vi "set_positions.vi"(7 "PicoMotor (in)":refnum<class "PicoMotor.lvclass">, 8 "error IO":errorcluster, 10 "enables":bool[](array[boolean]), 11 "set positions":i32[](array[numeric])) -> (0 "error out":errorcluster, 3 "PicoMotor":refnum<class "PicoMotor.lvclass">)   [LabVIEW 2013, in "PicoMotor.lvclass"]
uses:
  PicoMotor.lvclass
  PicoMotor.lvclass/PicoMotor.ctl
  Globals.vi
panel:
  out "enableds":bool[](array[boolean])
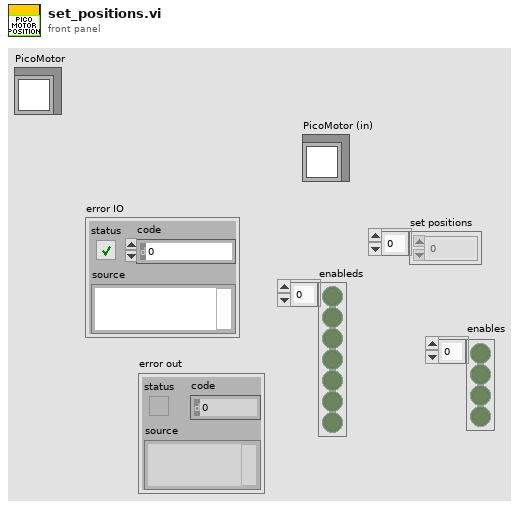
[diagram p1: front panel]
types:
  T1 = typedef "Experiment.lvclass/states.ctl" = enum16{"run", "pause", "shutdown gracefully", "halt immediately", "waiting for connection", "waiting for command"}
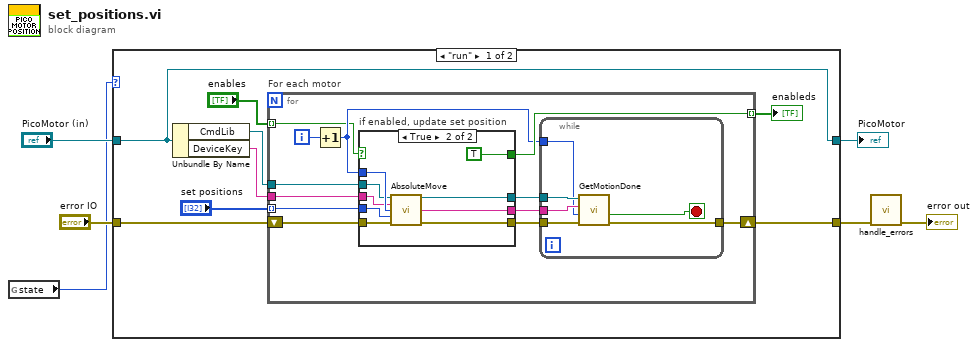
[diagram p0: block diagram]
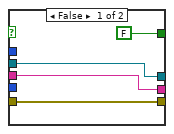
[diagram p2: hidden frame]
diagram:
  n1 = global read "Globals.vi" "state"() -> (w1:T1)
  n2 = case shown="\"run\"" w1 {
    tunnel: [w13 w47] -> w6
    tunnel: "error IO" -> [w14 w47]
    tunnel: "PicoMotor (in)" -> [w7 w46]
    tunnel: [w7 w46] -> w2
    frame "run" {
      n3 = Unbundle By Name(w7) -> ("CmdLib"=w9:refnum<k24>, "DeviceKey"=w8:string)
      n4 = for "For each motor" {
        shift-right: [w17] -> w13
        shift-left: w14 -> [w25]
        tunnel: w9 -> [w23]
        tunnel: w8 -> [w24]
        tunnel: "set positions" -> [w21] mode=indexing
        tunnel: [w22] -> w11 mode=indexing
        tunnel: "enables" -> [w15] mode=indexing
        i -> [w26]
        n5 = Increment(x=w26) -> (x+1=w16:i32)
        n6 = case "if enabled, update set position" shown="True" w15 {
          tunnel: w24 -> [w34 w40]
          tunnel: w25 -> [w36 w42]
          tunnel: w23 -> [w33 w39]
          tunnel: w16 -> [_ w45]
          tunnel: [w36 w41] -> w18
          tunnel: w21 -> [_ w43]
          tunnel: [FALSE TRUE] -> w22
          tunnel: [w34 w38] -> w20
          tunnel: [w33 w37] -> w19
          frame False {
          }
          frame True {
            n7 = call "AbsoluteMove.vi"("CmdLib In"=w39, "DeviceKey In"=w40, "Motor"=w45, "Target Pos"=w43, "error in (no error)"=w42) -> ("CmdLib Out"=w37:refnum<k24>, "DeviceKey Out"=w38:string, "error out"=w41:errorcluster)  [unwired: 8 in]
          }
        }
        n8 = while {
          tunnel: w20 -> [w32]
          tunnel: w19 -> [w31]
          tunnel: w18 -> [w30]
          tunnel: [w29] -> w17
          tunnel: w16 -> [w27]
          stop <- w28 stop-if-true
          n9 = call "GetMotionDone.vi"("error in (no error)"=w30, "Motor"=w27, "DeviceKey In"=w32, "CmdLib In"=w31) -> ("error out"=w29:errorcluster, "Is Motion Done"=w28:bool)  [unwired: 2 out]
        }
      }
      "enableds" <- w11
    }
    frame Default {
    }
  }
  "PicoMotor" <- w2
  n10 = call "handle_errors.vi"("error in (no error)"=w6) -> ("error out"=→"error out":errorcluster)  [unwired: 14 in]
